vi "oa_Get DSA Oversample Rate and Filter Delay.vi"(10 "sample rate":dbl, 11 "device info":T1 {"DSA device type" items=["Custom"=0, "4472"=1, "4474"=11, "4461"=2, "4462"=12, "4464"=13, "449x"=7, "9232"=8, "9233"=3, "9234"=4, "9229"=5, "9239"=6]}) -> (2 "SampClkTimebase":dbl, 3 "input delay":dbl)   [LabVIEW 2017, in "SoundVib_TachProcess.lvlib"]
uses:
  <vilib>/addons/Sound and Vibration/Order Analysis/Tach Process/SoundVib_TachProcess.lvlib
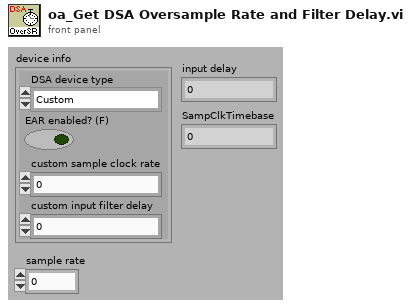
[diagram p1: front panel]
types:
  T1 = cluster{"DSA device type":u16, "EAR enabled? (F)":bool, "custom sample clock rate":dbl, "custom input filter delay":dbl}
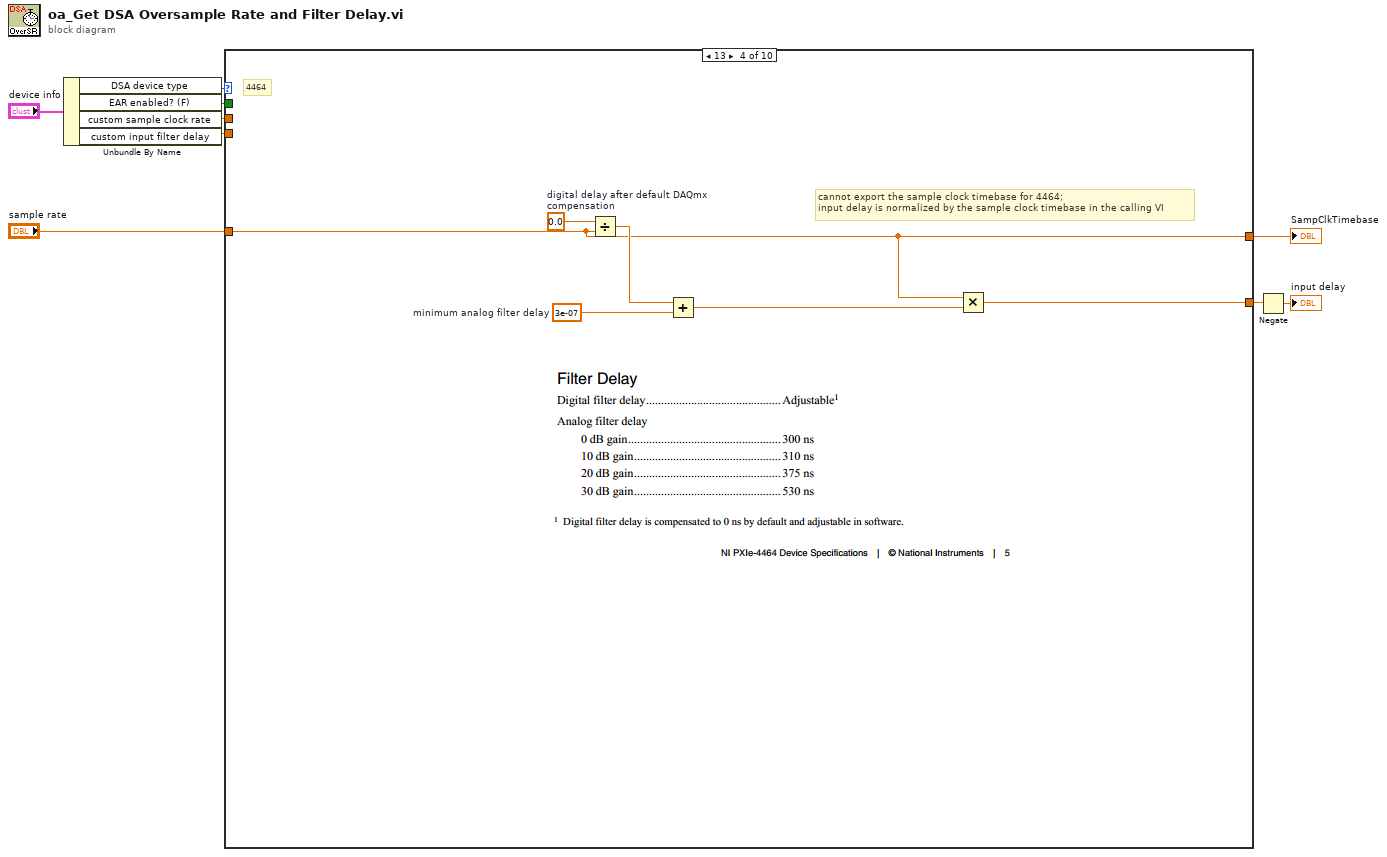
[diagram p0: block diagram]
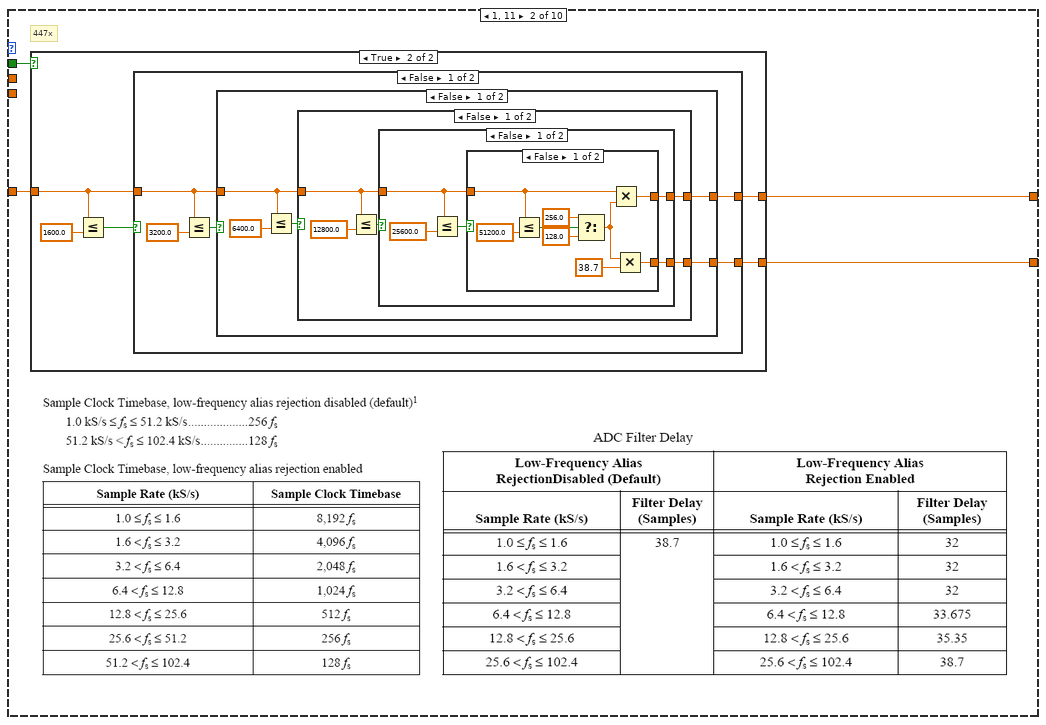
[diagram p3: hidden frame]
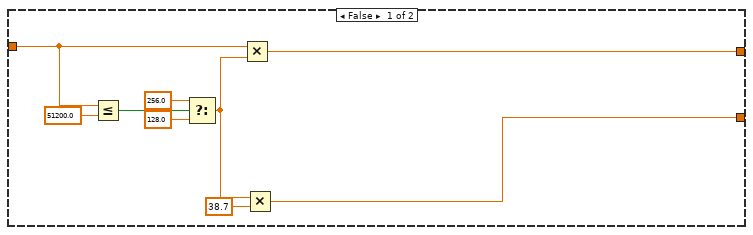
[diagram p4: hidden frame]
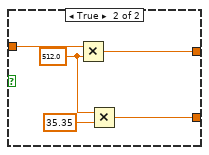
[diagram p5: hidden frame]
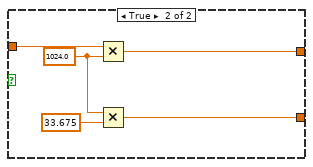
[diagram p6: hidden frame]
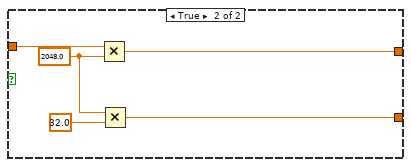
[diagram p7: hidden frame]
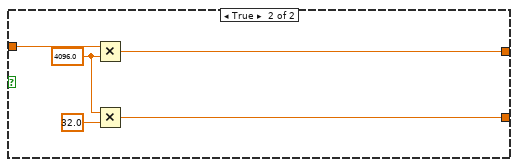
[diagram p8: hidden frame]
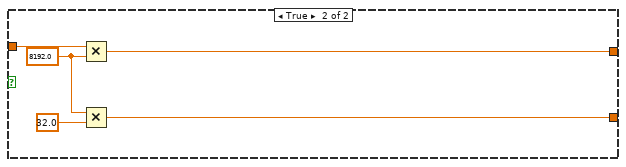
[diagram p9: hidden frame]
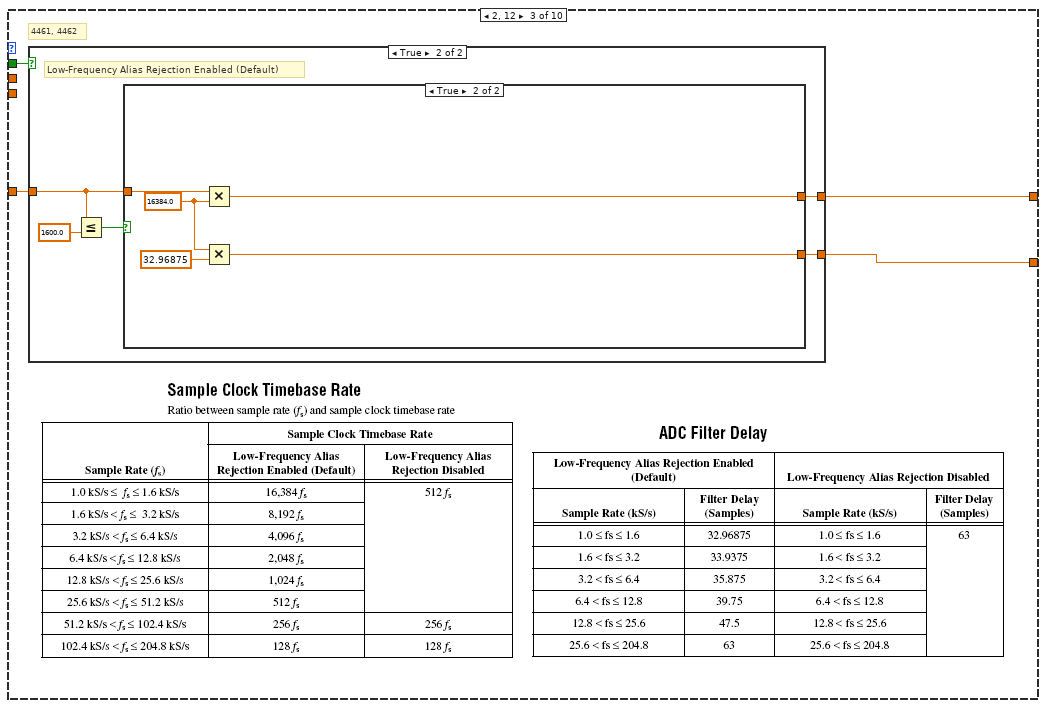
[diagram p10: hidden frame]
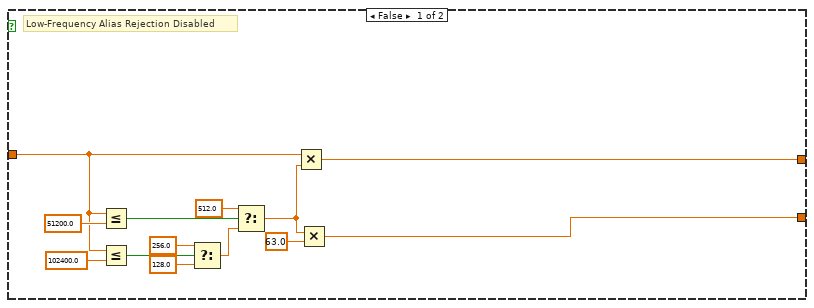
[diagram p11: hidden frame]
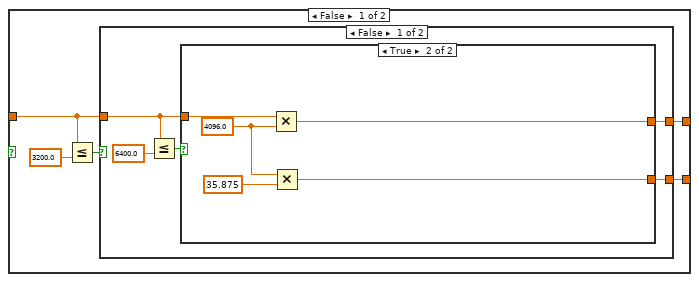
[diagram p12: hidden frame]
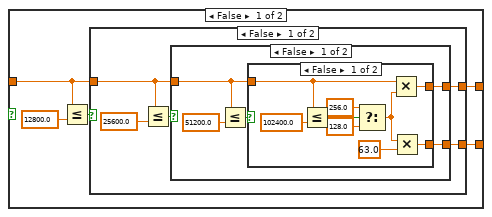
[diagram p13: hidden frame]
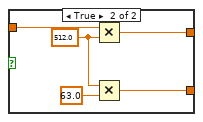
[diagram p14: hidden frame]
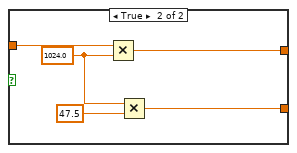
[diagram p15: hidden frame]
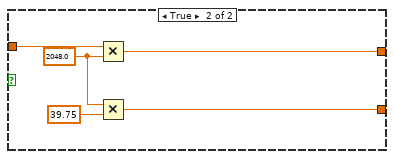
[diagram p16: hidden frame]
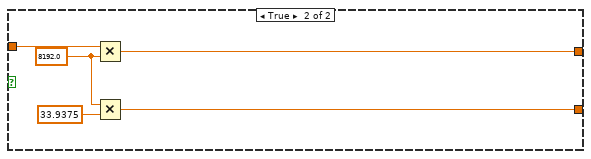
[diagram p17: hidden frame]
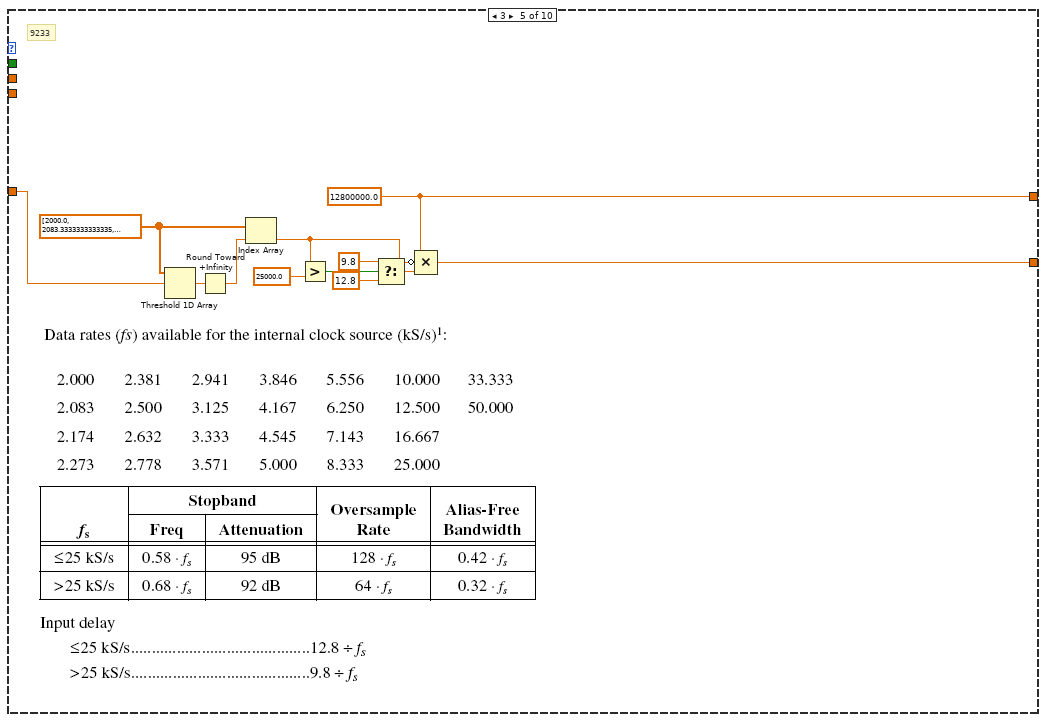
[diagram p18: hidden frame]
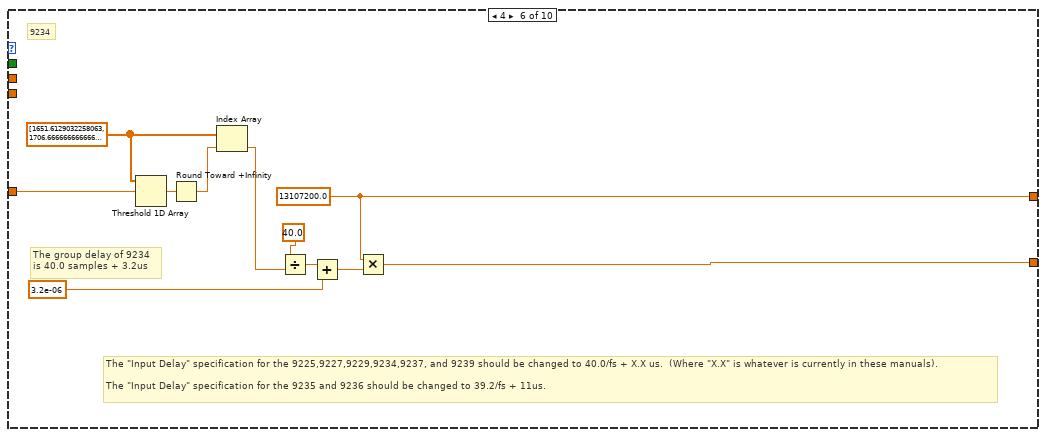
[diagram p19: hidden frame]
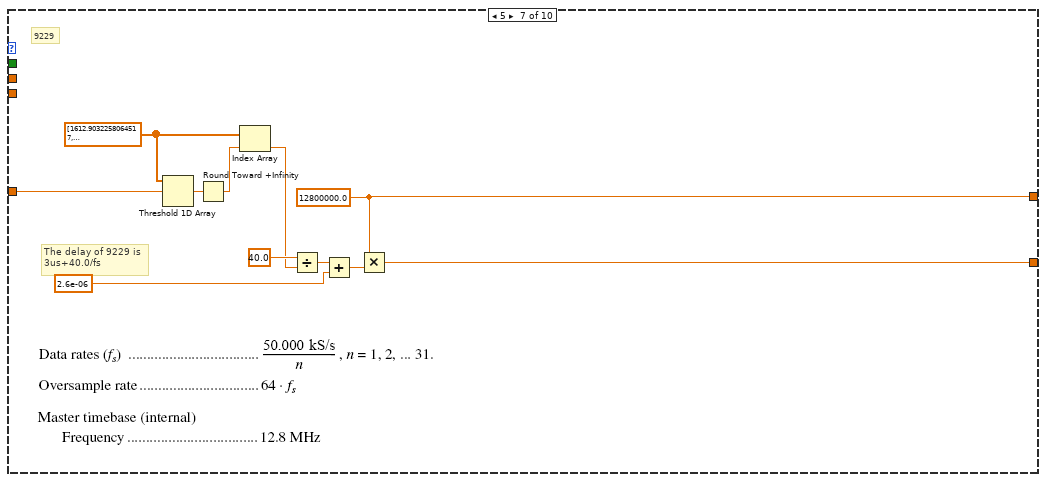
[diagram p20: hidden frame]
diagram:
  n1 = Unbundle By Name("device info") -> ("DSA device type"=w8:u16, "EAR enabled? (F)"=w7:bool, "custom sample clock rate"=w6:dbl, "custom input filter delay"=w5:dbl)
  n2 = case shown="13" w8 {
    tunnel: "sample rate" -> [_ w15 w87 w170 w178 w191 w202 w213 w222 w343]
    tunnel: [w10 w12 w84 w171 w176 w188 w199 w210 w223 w344] -> w3
    tunnel: [w11 w13 w85 w170 w177 w189 w200 w212 w224 w342] -> w2
    tunnel: w6 -> [w11 _ _ _ _ _ _ _ _ _]
    tunnel: w7 -> [_ w14 w86 _ _ _ _ _ w221 _]
    tunnel: w5 -> [w10 _ _ _ _ _ _ _ _ _]
    frame 0, Default {
    }
    frame 1, 11 {
      # "447x"
      n3 = case shown="True" w14 {
        tunnel: w15 -> [w18 w27]
        tunnel: [w19 w25] -> w12
        tunnel: [w16 w26] -> w13
        frame False {
          n4 = Less Or Equal?(x=w18, y=51200.0) -> (x <= y?=w23:bool)
          n5 = Select(t=256.0, s=w23, f=128.0) -> (s? t:f=w17:dbl)
          n6 = Multiply(x=w18, y=w17) -> (x*y=w16:dbl)
          n7 = Multiply(x=w17, y=38.7) -> (x*y=w19:dbl)
        }
        frame True {
          n8 = Less Or Equal?(x=w27, y=1600.0) -> (x <= y?=w28:bool)
          n9 = case shown="False" w28 {
            tunnel: w27 -> [w32 w83]
            tunnel: [w31 w82] -> w26
            tunnel: [w30 w79] -> w25
            frame False {
              n10 = Less Or Equal?(x=w32, y=3200.0) -> (x <= y?=w33:bool)
              n11 = case shown="False" w33 {
                tunnel: w32 -> [w37 w78]
                tunnel: [w36 w77] -> w31
                tunnel: [w35 w74] -> w30
                frame False {
                  n12 = Less Or Equal?(x=w37, y=6400.0) -> (x <= y?=w38:bool)
                  n13 = case shown="False" w38 {
                    tunnel: w37 -> [w42 w73]
                    tunnel: [w41 w71] -> w36
                    tunnel: [w40 w69] -> w35
                    frame False {
                      n14 = Less Or Equal?(x=w42, y=12800.0) -> (x <= y?=w43:bool)
                      n15 = case shown="False" w43 {
                        tunnel: w42 -> [w47 w68]
                        tunnel: [w46 w67] -> w41
                        tunnel: [w45 w64] -> w40
                        frame False {
                          n16 = Less Or Equal?(x=w47, y=25600.0) -> (x <= y?=w48:bool)
                          n17 = case shown="False" w48 {
                            tunnel: w47 -> [w53 w63]
                            tunnel: [w54 w62] -> w46
                            tunnel: [w51 w59] -> w45
                            frame False {
                              n18 = Less Or Equal?(x=w53, y=51200.0) -> (x <= y?=w57:bool)
                              n19 = Select(t=256.0, s=w57, f=128.0) -> (s? t:f=w52:dbl)
                              n20 = Multiply(x=w53, y=w52) -> (x*y=w54:dbl)
                              n21 = Multiply(x=w52, y=38.7) -> (x*y=w51:dbl)
                            }
                            frame True {
                              w61 = 512.0 ("y")
                              n22 = Multiply(x=w63, y=w61) -> (x*y=w62:dbl)
                              n23 = Multiply(x=w61, y=35.35) -> (x*y=w59:dbl)
                            }
                          }
                        }
                        frame True {
                          w66 = 1024.0 ("y")
                          n24 = Multiply(x=w68, y=w66) -> (x*y=w67:dbl)
                          n25 = Multiply(x=w66, y=33.675) -> (x*y=w64:dbl)
                        }
                      }
                    }
                    frame True {
                      w70 = 2048.0 ("y")
                      n26 = Multiply(x=w73, y=w70) -> (x*y=w71:dbl)
                      n27 = Multiply(x=w70, y=32.0) -> (x*y=w69:dbl)
                    }
                  }
                }
                frame True {
                  w76 = 4096.0 ("y")
                  n28 = Multiply(x=w78, y=w76) -> (x*y=w77:dbl)
                  n29 = Multiply(x=w76, y=32.0) -> (x*y=w74:dbl)
                }
              }
            }
            frame True {
              w81 = 8192.0 ("y")
              n30 = Multiply(x=w83, y=w81) -> (x*y=w82:dbl)
              n31 = Multiply(x=w81, y=32.0) -> (x*y=w79:dbl)
            }
          }
        }
      }
    }
    frame 2, 12 {
      # "4461, 4462"
      n32 = case shown="True" w86 {
        tunnel: w87 -> [w94 w103]
        tunnel: [w96 w101] -> w84
        tunnel: [w95 w102] -> w85
        frame False {
          # "Low-Frequency Alias Rejection Disabled"
          n33 = Less Or Equal?(x=w94, y=51200.0) -> (x <= y?=w99:bool)
          n34 = Less Or Equal?(x=w94, y=102400.0) -> (x <= y?=w92:bool)
          n35 = Select(t=256.0, s=w92, f=128.0) -> (s? t:f=w89:dbl)
          n36 = Select(t=512.0, s=w99, f=w89) -> (s? t:f=w88:dbl)
          n37 = Multiply(x=w94, y=w88) -> (x*y=w95:dbl)
          n38 = Multiply(x=w88, y=63.0) -> (x*y=w96:dbl)
        }
        frame True {
          # "Low-Frequency Alias Rejection Enabled (Default)"
          n39 = Less Or Equal?(x=w103, y=1600.0) -> (x <= y?=w104:bool)
          n40 = case shown="True" w104 {
            tunnel: w103 -> [w108 w169]
            tunnel: [w107 w168] -> w102
            tunnel: [w106 w165] -> w101
            frame False {
              n41 = Less Or Equal?(x=w108, y=3200.0) -> (x <= y?=w109:bool)
              n42 = case shown="False" w109 {
                tunnel: w108 -> [w113 w164]
                tunnel: [w112 w163] -> w107
                tunnel: [w111 w160] -> w106
                frame False {
                  n43 = Less Or Equal?(x=w113, y=6400.0) -> (x <= y?=w114:bool)
                  n44 = case shown="True" w114 {
                    tunnel: w113 -> [w118 w159]
                    tunnel: [w117 w157] -> w112
                    tunnel: [w116 w155] -> w111
                    frame False {
                      n45 = Less Or Equal?(x=w118, y=12800.0) -> (x <= y?=w119:bool)
                      n46 = case shown="False" w119 {
                        tunnel: w118 -> [w123 w154]
                        tunnel: [w122 w153] -> w117
                        tunnel: [w121 w150] -> w116
                        frame False {
                          n47 = Less Or Equal?(x=w123, y=25600.0) -> (x <= y?=w124:bool)
                          n48 = case shown="False" w124 {
                            tunnel: w123 -> [w128 w149]
                            tunnel: [w127 w148] -> w122
                            tunnel: [w126 w145] -> w121
                            frame False {
                              n49 = Less Or Equal?(x=w128, y=51200.0) -> (x <= y?=w129:bool)
                              n50 = case shown="False" w129 {
                                tunnel: w128 -> [w135 w144]
                                tunnel: [w134 w143] -> w127
                                tunnel: [w133 w140] -> w126
                                frame False {
                                n51 = Less Or Equal?(x=w135, y=102400.0) -> (x <= y?=w138:bool)
                                n52 = Select(t=256.0, s=w138, f=128.0) -> (s? t:f=w132:dbl)
                                n53 = Multiply(x=w135, y=w132) -> (x*y=w134:dbl)
                                n54 = Multiply(x=w132, y=63.0) -> (x*y=w133:dbl)
                                }
                                frame True {
                                w142 = 512.0 ("y")
                                n55 = Multiply(x=w144, y=w142) -> (x*y=w143:dbl)
                                n56 = Multiply(x=w142, y=63.0) -> (x*y=w140:dbl)
                                }
                              }
                            }
                            frame True {
                              w147 = 1024.0 ("y")
                              n57 = Multiply(x=w149, y=w147) -> (x*y=w148:dbl)
                              n58 = Multiply(x=w147, y=47.5) -> (x*y=w145:dbl)
                            }
                          }
                        }
                        frame True {
                          w152 = 2048.0 ("y")
                          n59 = Multiply(x=w154, y=w152) -> (x*y=w153:dbl)
                          n60 = Multiply(x=w152, y=39.75) -> (x*y=w150:dbl)
                        }
                      }
                    }
                    frame True {
                      w156 = 4096.0 ("y")
                      n61 = Multiply(x=w159, y=w156) -> (x*y=w157:dbl)
                      n62 = Multiply(x=w156, y=35.875) -> (x*y=w155:dbl)
                    }
                  }
                }
                frame True {
                  w162 = 8192.0 ("y")
                  n63 = Multiply(x=w164, y=w162) -> (x*y=w163:dbl)
                  n64 = Multiply(x=w162, y=33.9375) -> (x*y=w160:dbl)
                }
              }
            }
            frame True {
              w167 = 16384.0 ("y")
              n65 = Multiply(x=w169, y=w167) -> (x*y=w168:dbl)
              n66 = Multiply(x=w167, y=32.96875) -> (x*y=w165:dbl)
            }
          }
        }
      }
    }
    frame 13 {
      w175 = 0.0  # digital delay after default DAQmx compensation
      w173 = 3e-07  # minimum analog filter delay
      # "cannot export the sample clock timebase for 4464;\ninput delay is normalized by the sample clock timebase in the calling VI"
      # "4464"
      n67 = Divide(x=w175, y=w170) -> (x/y=w174:dbl)
      n68 = Add(x=w174, y=w173) -> (x+y=w172:dbl)
      n69 = Multiply(x=w170, y=w172) -> (x*y=w171:dbl)
    }
    frame 3 {
      w177 = 12800000.0 ("SampClkTimebase")
      w180 = dbl[] [2000.0, 2083.3333333333335, 2173.913043478261, 2272.7272727272725, 2380.9523809523807, 2500.0, 2631.5789473684213, 2777.777777777778, 2941.176470588235, 3125.0, 3333.3333333333335, 3571.4285714285716, 3846.153846153846, 4166.666666666667, 4545.454545454545, 5000.0, 5555.555555555556, 6250.0, 7142.857142857143, 8333.333333333334, 10000.0, 12500.0, 16666.666666666668, 25000.0, 33333.333333333336, 50000.0] ("reversed array")
      # "9233"
      n70 = Threshold 1D Array(2:w178, 3:w180) -> (0:w187:dbl)  [unwired: 1 in]
      n71 = Round Toward +Infinity(x=w187) -> (ceil(x): smallest int >= x=w186:dbl)
      n72 = Index Array(array=w180, index=w186) -> (element=w179:dbl)
      n73 = Greater?(x=w179, y=25000.0) -> (0:w184:bool)
      n74 = Select(t=9.8, s=w184, f=12.8) -> (s? t:f=w181:dbl)
      n75 = Compound Arithmetic op=MULTIPLY(w177, invert w179, w181) -> (w176:dbl)
    }
    frame 4 {
      w189 = 13107200.0 ("SampClkTimebase")
      w196 = dbl[] [1651.6129032258063, 1706.6666666666667, 1765.5172413793102, 1828.5714285714287, 1896.2962962962963, 1969.2307692307693, 2048.0, 2133.3333333333335, 2226.086956521739, 2327.2727272727275, 2438.095238095238, 2560.0, 2694.7368421052633, 2844.4444444444443, 3011.764705882353, 3200.0, 3413.3333333333335, 3657.1428571428573, 3938.4615384615386, 4266.666666666667, 4654.545454545455, 5120.0, 5688.888888888889, 6400.0, 7314.285714285715, 8533.333333333334, 10240.0, 12800.0, 17066.666666666668, 25600.0, 51200.0] ("Array")
      # "The \"Input Delay\" specification for the 9225,9227,9229,9234,9237, and 9239 should be changed to 40.0/fs + X.X us.  (Where \"X.X\" is whatever is currently in these manuals).\n\nThe \"Input Delay\" specification for the 9235 and 9236 should be changed to 39.2/fs + 11us."
      # "The group delay of 9234\nis 40.0 samples + 3.2us"
      # "9234"
      n76 = Threshold 1D Array(2:w191, 3:w196) -> (0:w197:dbl)  [unwired: 1 in]
      n77 = Round Toward +Infinity(x=w197) -> (ceil(x): smallest int >= x=w198:dbl)
      n78 = Index Array(array=w196, index=w198) -> (element=w193:dbl)
      n79 = Divide(x=40.0 ("y"), y=w193) -> (x/y=w194:dbl)
      n80 = Add(x=w194, y=3.2e-06) -> (x+y=w190:dbl)
      n81 = Multiply(x=w189, y=w190) -> (x*y=w188:dbl)
    }
    frame 5 {
      w207 = dbl[] [1612.9032258064517, 1666.6666666666667, 1724.1379310344828, 1785.7142857142858, 1851.851851851852, 1923.076923076923, 2000.0, 2083.3333333333335, 2173.913043478261, 2272.7272727272725, 2380.9523809523807, 2500.0, 2631.5789473684213, 2777.777777777778, 2941.176470588235, 3125.0, 3333.3333333333335, 3571.4285714285716, 3846.153846153846, 4166.666666666667, 4545.454545454545, 5000.0, 5555.555555555556, 6250.0, 7142.857142857143, 8333.333333333334, 10000.0, 12500.0, 16666.666666666668, 25000.0, 50000.0] ("reversed array")
      w200 = 12800000.0 ("y")
      # "The delay of 9229 is\n3us+40.0/fs"
      # "9229"
      n82 = Threshold 1D Array(2:w202, 3:w207) -> (0:w209:dbl)  [unwired: 1 in]
      n83 = Round Toward +Infinity(x=w209) -> (ceil(x): smallest int >= x=w208:dbl)
      n84 = Index Array(array=w207, index=w208) -> (element=w204:dbl)
      n85 = Divide(x=40.0 ("y"), y=w204) -> (x/y=w203:dbl)
      n86 = Add(x=w203, y=2.6e-06) -> (x+y=w201:dbl)
      n87 = Multiply(x=w200, y=w201) -> (x*y=w199:dbl)
    }
    frame 6 {
      w218 = dbl[] [1612.9032258064517, 1666.6666666666667, 1724.1379310344828, 1785.7142857142858, 1851.851851851852, 1923.076923076923, 2000.0, 2083.3333333333335, 2173.913043478261, 2272.7272727272725, 2380.9523809523807, 2500.0, 2631.5789473684213, 2777.777777777778, 2941.176470588235, 3125.0, 3333.3333333333335, 3571.4285714285716, 3846.153846153846, 4166.666666666667, 4545.454545454545, 5000.0, 5555.555555555556, 6250.0, 7142.857142857143, 8333.333333333334, 10000.0, 12500.0, 16666.666666666668, 25000.0, 50000.0] ("reversed array")
      w212 = 12800000.0 ("y")
      # "The delay of 9239 is\n3us+40.0/fs"
      # "9239"
      n88 = Threshold 1D Array(2:w213, 3:w218) -> (0:w220:dbl)  [unwired: 1 in]
      n89 = Round Toward +Infinity(x=w220) -> (ceil(x): smallest int >= x=w219:dbl)
      n90 = Index Array(array=w218, index=w219) -> (element=w215:dbl)
      n91 = Divide(x=40.0 ("y"), y=w215) -> (x/y=w214:dbl)
      n92 = Add(x=w214, y=3e-06) -> (x+y=w211:dbl)
      n93 = Multiply(x=w212, y=w211) -> (x*y=w210:dbl)
    }
    frame 7 {
      # "100 <=   fs  <= 200   \t131072 fs\n200 <      fs  <= 400\t\t  65536 fs\n400 <      fs  <= 800\t\t  32768 fs\n800 <      fs  <= 1600\t\t16384 fs"
      # "449x"
      n94 = case shown="True" w221 {
        tunnel: w222 -> [w231 w244]
        tunnel: [w238 w242] -> w223
        tunnel: [w237 w243] -> w224
        frame False {
          # "Low-Frequency Alias Rejection Disabled (Default)"
          n95 = Less Or Equal?(x=w231, y=51200.0) -> (x <= y?=w240:bool)
          n96 = Less Or Equal?(x=w231, y=102400.0) -> (x <= y?=w235:bool)
          n97 = Less?(x=w231, y=1000.0) -> (x < y?=w228:bool)
          n98 = Select(t=256.0, s=w235, f=128.0) -> (s? t:f=w229:dbl)
          n99 = Select(t=0.0, s=w228, f=63.0) -> (s? t:f=w225:dbl)
          n100 = Select(t=512.0, s=w240, f=w229) -> (s? t:f=w232:dbl)
          n101 = Multiply(x=w231, y=w232) -> (x*y=w237:dbl)
          n102 = Multiply(x=w232, y=w225) -> (x*y=w238:dbl)
        }
        frame True {
          # "Low-Frequency Alias Rejection Enabled"
          n103 = Less Or Equal?(x=w244, y=200.0) -> (x <= y?=w245:bool)
          n104 = case shown="False" w245 {
            tunnel: w244 -> [w249 w340]
            tunnel: [w248 w339] -> w243
            tunnel: [w247 w336] -> w242
            frame False {
              n105 = Less Or Equal?(x=w249, y=400.0) -> (x <= y?=w250:bool)
              n106 = case shown="True" w250 {
                tunnel: w249 -> [w254 w335]
                tunnel: [w253 w334] -> w248
                tunnel: [w252 w331] -> w247
                frame False {
                  n107 = Less Or Equal?(x=w254, y=800.0) -> (x <= y?=w255:bool)
                  n108 = case shown="False" w255 {
                    tunnel: w254 -> [w259 w330]
                    tunnel: [w258 w328] -> w253
                    tunnel: [w257 w326] -> w252
                    frame False {
                      n109 = Less Or Equal?(x=w259, y=1600.0) -> (x <= y?=w260:bool)
                      n110 = case shown="False" w260 {
                        tunnel: w259 -> [w264 w325]
                        tunnel: [w263 w324] -> w258
                        tunnel: [w262 w321] -> w257
                        frame False {
                          n111 = Less Or Equal?(x=w264, y=3200.0) -> (x <= y?=w265:bool)
                          n112 = case shown="False" w265 {
                            tunnel: w264 -> [w269 w320]
                            tunnel: [w268 w319] -> w263
                            tunnel: [w267 w316] -> w262
                            frame False {
                              n113 = Less Or Equal?(x=w269, y=6400.0) -> (x <= y?=w270:bool)
                              n114 = case shown="False" w270 {
                                tunnel: w269 -> [w274 w315]
                                tunnel: [w273 w314] -> w268
                                tunnel: [w272 w311] -> w267
                                frame False {
                                n115 = Less Or Equal?(x=w274, y=12800.0) -> (x <= y?=w275:bool)
                                n116 = case shown="False" w275 {
                                tunnel: w274 -> [w280 w310]
                                tunnel: [w278 w307] -> w273
                                tunnel: [w277 w306] -> w272
                                frame False {
                                n117 = Less Or Equal?(x=w280, y=25600.0) -> (x <= y?=w279:bool)
                                n118 = case shown="False" w279 {
                                tunnel: w280 -> [w284 w305]
                                tunnel: [w283 w304] -> w278
                                tunnel: [w282 w302] -> w277
                                frame False {
                                n119 = Less Or Equal?(x=w284, y=51200.0) -> (x <= y?=w285:bool)
                                n120 = case shown="True" w285 {
                                tunnel: w284 -> [w290 w300]
                                tunnel: [w291 w299] -> w283
                                tunnel: [w289 w296] -> w282
                                frame False {
                                n121 = Less Or Equal?(x=w290, y=102.4) -> (x <= y?=w294:bool)
                                n122 = Select(t=256.0, s=w294, f=128.0) -> (s? t:f=w288:dbl)
                                n123 = Multiply(x=w290, y=w288) -> (x*y=w291:dbl)
                                n124 = Multiply(x=w288, y=63.0) -> (x*y=w289:dbl)
                                }
                                frame True {
                                w298 = 512.0 ("y")
                                n125 = Multiply(x=w300, y=w298) -> (x*y=w299:dbl)
                                n126 = Multiply(x=w298, y=63.0) -> (x*y=w296:dbl)
                                }
                                }
                                }
                                frame True {
                                w303 = 1024.0 ("y")
                                n127 = Multiply(x=w305, y=w303) -> (x*y=w304:dbl)
                                n128 = Multiply(x=w303, y=47.5) -> (x*y=w302:dbl)
                                }
                                }
                                }
                                frame True {
                                w309 = 2048.0 ("y")
                                n129 = Multiply(x=w310, y=w309) -> (x*y=w307:dbl)
                                n130 = Multiply(x=w309, y=39.75) -> (x*y=w306:dbl)
                                }
                                }
                                }
                                frame True {
                                w313 = 4096.0 ("y")
                                n131 = Multiply(x=w315, y=w313) -> (x*y=w314:dbl)
                                n132 = Multiply(x=w313, y=35.88) -> (x*y=w311:dbl)
                                }
                              }
                            }
                            frame True {
                              w318 = 8192.0 ("y")
                              n133 = Multiply(x=w320, y=w318) -> (x*y=w319:dbl)
                              n134 = Multiply(x=w318, y=33.94) -> (x*y=w316:dbl)
                            }
                          }
                        }
                        frame True {
                          w323 = 16384.0 ("y")
                          n135 = Multiply(x=w325, y=w323) -> (x*y=w324:dbl)
                          n136 = Multiply(x=w323, y=32.97) -> (x*y=w321:dbl)
                        }
                      }
                    }
                    frame True {
                      w327 = 32768.0 ("y")
                      n137 = Multiply(x=w330, y=w327) -> (x*y=w328:dbl)
                      n138 = Multiply(x=w327, y=32.48) -> (x*y=w326:dbl)
                    }
                  }
                }
                frame True {
                  w333 = 65536.0 ("y")
                  n139 = Multiply(x=w335, y=w333) -> (x*y=w334:dbl)
                  n140 = Multiply(x=w333, y=32.24) -> (x*y=w331:dbl)
                }
              }
            }
            frame True {
              w338 = 131072.0 ("y")
              n141 = Multiply(x=w340, y=w338) -> (x*y=w339:dbl)
              n142 = Multiply(x=w338, y=32.12) -> (x*y=w336:dbl)
            }
          }
        }
      }
    }
    frame 8 {
      # "9232"
      n143 = call <vilib>:"oa_Get DSA 9232 Oversample Rate and Filter Delay.vi"("Requested Sample Rate"=w343) -> ("Input Delay"=w341:dbl, "Internal Master Timebase"=w342:dbl)  [unwired: 7 in, 2 out]
      n144 = Multiply(x=w342, y=w341) -> (x*y=w344:dbl)
    }
  }
  "SampClkTimebase" <- w2
  n145 = Negate(x=w3) -> (-x=→"input delay":dbl)
